vi "Post-Build Action Post Pre Install.vi"(5 "Files Generated by Build":path[](array[path]), 6 "Top Level/Always Included VIs":path[](array[path]), 7 "Destination Path":path, 8 "error in (no error)":errorcluster, 9 "Target Name":string, 10 "Build Specification Name":string, 11 "Project Path":path) -> (0 "error out":errorcluster)   [LabVIEW 2015, in "veristand-steps-build-tools.lvlib"]
uses:
  veristand-steps-build-tools.lvlib
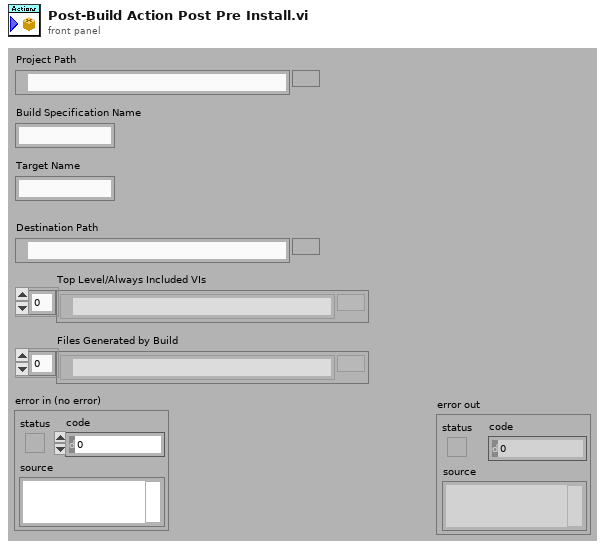
[diagram p1: front panel]
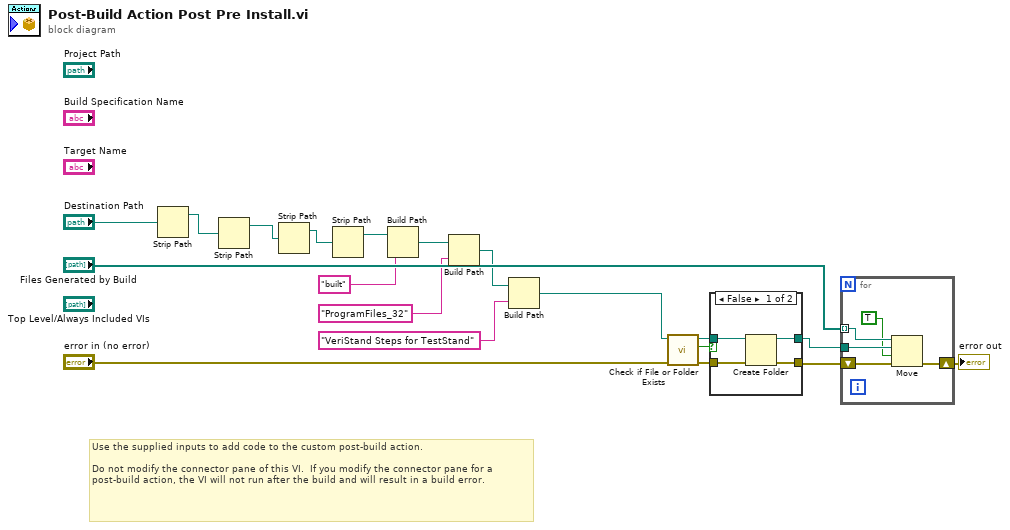
[diagram p0: block diagram]
diagram:
  # "Use the supplied inputs to add code to the custom post-build action.\n\nDo not modify the connector pane of this VI.  If you modify the connector pane for a post-build action, the VI will not run after the build and will result in a build error."
  n1 = Strip Path(path="Destination Path") -> (stripped path=w10:path)  [unwired: 1 out]
  n2 = Strip Path(path=w10) -> (stripped path=w9:path)  [unwired: 1 out]
  n3 = Strip Path(path=w9) -> (stripped path=w8:path)  [unwired: 1 out]
  n4 = Strip Path(path=w8) -> (stripped path=w7:path)  [unwired: 1 out]
  n5 = Build Path(base path=w7, name or relative path="built") -> (appended path=w5:path)
  n6 = Build Path(base path=w5, name or relative path="ProgramFiles_32") -> (appended path=w3:path)
  n7 = Build Path(base path=w3, name or relative path="VeriStand Steps for TestStand") -> (appended path=w1:path)
  n8 = call <vilib>:"Check if File or Folder Exists.vi"("error in (no error)"="error in (no error)", "path"=w1) -> ("error out"=w18:errorcluster, "file or folder exists?"=w17:bool, "dup path"=w16:path)  [unwired: 7 in]
  n9 = case shown="False" w17 {
    tunnel: w18 -> [w23 w24]
    tunnel: w16 -> [w21 w25]
    tunnel: [w22 w24] -> w15
    tunnel: [w20 w25] -> w13
    frame False {
      n10 = Create Folder(path (use dialog)=w21, error in=w23) -> (created path=w20:path, error out=w22:errorcluster)  [unwired: 1 in, 1 out]
    }
    frame True {
    }
  }
  n11 = for {
    tunnel: w13 -> [w28]
    shift-right: [w29] -> w14
    shift-left: w15 -> [w30]
    tunnel: "Files Generated by Build" -> [w27] mode=indexing
    n12 = Move(source path=w27, error in=w30, 9:TRUE ("overwrite (F)"), 10:w28) -> (error out=w29:errorcluster)  [unwired: 1 in, 2 out]
  }
  "error out" <- w14
